vi "Read Tag Description.vi"(8 "error in (no error)":errorcluster, 11 "Tag Name":string) -> (0 "error out":errorcluster, 3 "Description":string)   [LabVIEW 2020, in "Current Value Table(Rebuild).lvlib"]
doc: "This VI will retrieve the description of a single tag. It can be easily modified to retrieve descriptions for a group of tags."
uses:
  FGVs/Tag Memory Methods.ctl
  Current Value Table(Rebuild).lvlib
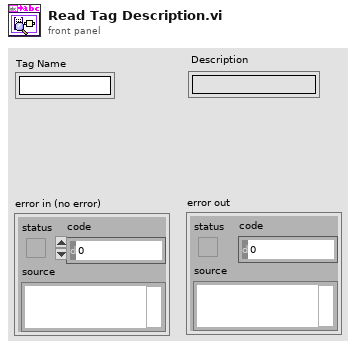
[diagram p1: front panel]
types:
  T1 = typedef "Current Value Table(Rebuild).lvlib/Tag Memory Methods.ctl" = enum16{"Clear", "Read Tag Index", "Read Tag Indices", "Generate Group", "Add Tag", "Overwrite Tag", "Read Description", "Get Stored Tags", "Write Description"}
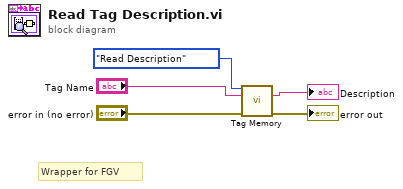
[diagram p0: block diagram]
diagram:
  # "Wrapper for FGV"
  n1 = call "Tag Memory.vi"("Method"=Tag_Memory_Methods."Read Description", "Tag"="Tag Name", "error in (no error)"="error in (no error)") -> ("Description"=→"Description":string, "error out"=→"error out":errorcluster)  [unwired: 7 in, 4 out]
